vi "Test Resize Greyscale.vi"(8 "error in (no error)":errorcluster, 11 "Test Case In":refnum<class "Image.lvclass">) -> (0 "error out":errorcluster, 3 "Test Case Out":refnum<class "Image.lvclass">)   [LabVIEW 2020, in "g_ar_toolkit.test.lvlib" / "Image.lvclass"]
uses:
  Image.lvclass
  C:/Program Files (x86)/National Instruments/LabVIEW 2020/vi.lib/Astemes/LUnit/Test Case.lvclass
  g_ar_toolkit.common/Image Size (Integer).ctl
  g_ar_toolkit.image/Interpolation Mode.ctl
  <vilib>/Astemes/LUnit/Test Case.lvclass/Test Case.ctl
  g_ar_toolkit.image/CreateEmptyImageGreyscale.vi
  g_ar_toolkit.image/ResizeGreyscale.vi
  4993e8ee-a06a-463a-9684-69129f64d5ce.vi
  g_ar_toolkit.image/Copy Array to Image.vi
  g_ar_toolkit.image/CopyArrayToImageGreyscale.vi
  g_ar_toolkit.image/CreateEmptyImageGreyscale.vi/6598b9e0-8a08-46f5-91fd-ca1b87217137.vi
  g_ar_toolkit.image/ResizeGreyscale.vi/eaa3f26c-b51e-4a69-9610-cf2aa5919b39.vi
  <vilib>/Astemes/LUnit/Append Pass Result.vi
  <vilib>/Astemes/LUnit/Append Fail Result.vi
  <vilib>/Astemes/LUnit/Describe Comparison.vi
  <vilib>/Astemes/LUnit/Compare Variants.vi
  g_ar_toolkit.image/CopyArrayToImageGreyscale.vi/26c70cee-9332-41f4-9755-08948a885cbe.vi
  <vilib>/Astemes/LUnit/Run In UI.vi
  <vilib>/Utility/error.llb/Clear Errors.vi
  g_ar_toolkit.common/Module Path.vi
  <vilib>/Utility/error.llb/Error Cluster From Error Code.vi
  <vilib>/picture/pixmap.llb/Flatten Pixmap.vi
  <vilib>/Astemes/LUnit/Describe Variant.vi
  Image.lvclass/Image.ctl
  g_ar_toolkit.image/g_ar_toolkit.image.lvlib
  g_ar_toolkit.common/g_ar_toolkit.common.lvlib
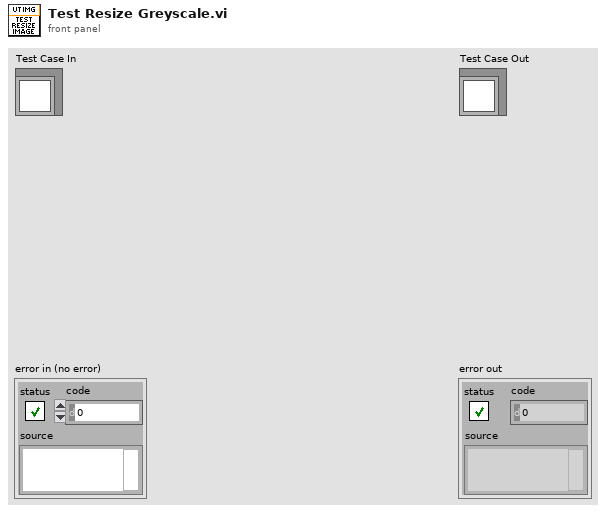
[diagram p1: front panel]
types:
  T1 = typedef "g_ar_toolkit.image.lvlib/Interpolation Mode.ctl" = enum8{"NEAREST", "LINEAR", "CUBIC", "AREA", "LANCZOS", "LINEAR_EXACT", "NEAREST_EXACT", "MAX"}
  T2 = typedef "g_ar_toolkit.common.lvlib/Image Size (Integer).ctl" = cluster{"Width":u16, "Height":u16}
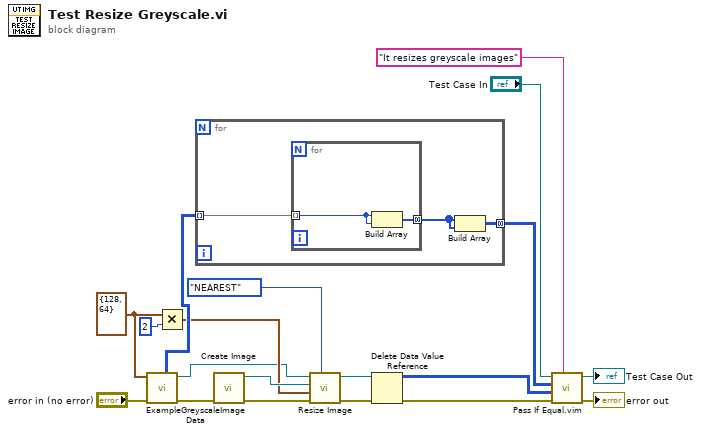
[diagram p0: block diagram]
diagram:
  w5 = T2 {"Width"=128, "Height"=64} ("Preallocated Image Size (Default - 0,0)")
  n1 = call "ExampleGreyscaleImageData.vi"("error in (no error)"="error in (no error)", "Image Size"=w5) -> ("error out"=w1:errorcluster, "Greyscale Destination Image"=w3:refnum<data-value>, "Greyscale Data"=w10:u8[][])  [unwired: 6 in, 1 out]
  n2 = Multiply(x=w5, y=u16 2) -> (x*y=w4:T2)
  n3 = for {
    tunnel: w10 -> [w22] mode=indexing
    tunnel: [w20] -> w9 mode=concatenating
    n4 = for {
      tunnel: w22 -> [w24] mode=indexing
      tunnel: [w23] -> w21 mode=concatenating
      n5 = Build Array(w24, w24) -> (w23:u8[])
    }
    n6 = Build Array(w21, w21) -> (w20:u8[][])
  }
  n7 = call-poly "Create Image.vi"("error in (no error)"=w1) -> ("error out"=w7:errorcluster, "New Greyscale Image"=w6:refnum<data-value>)  [unwired: 9 in]
  n8 = call-poly "Resize Image.vi"("Interpolation Mode (Default: CUBIC)"=Interpolation_Mode."NEAREST" ("OpenCV Interpolation Flag"), "error in (no error)"=w7, "New Image Size"=w4, "Greyscale Destination Image"=w6, "Greyscale Source Image"=w3) -> ("error out"=w12:errorcluster, "Greyscale Destination Image (duplicate)"=w13:refnum<data-value>)  [unwired: 5 in]
  n9 = Delete Data Value Reference(data value reference=w13, error in=w12) -> (data value=w14:u8[][], error out=w16:errorcluster)
  n10 = call "Pass If Equal.vim"("Description"="It resizes greyscale images", "error in (no error)"=w16, "Actual"=w14, "Expected"=w9, "LUnit Test Case In"="Test Case In") -> ("error out"=→"error out":errorcluster, "LUnit Test Case Out"=→"Test Case Out":refnum<class "Image.lvclass">)  [unwired: 5 in]
